vi "правый верхний(SubVI).vi"(10 "Width":u32, 11 "Height":u32) -> (2 "Numeric":u32, 3 "Numeric 2":u32)   [LabVIEW 2021]
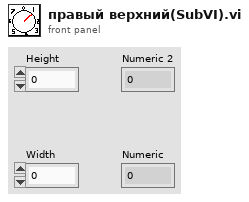
[diagram p1: front panel]
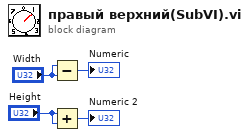
[diagram p0: block diagram]
diagram:
  n1 = Subtract(x="Width", y="Width") -> (x-y=→"Numeric":u32)
  n2 = Add(x="Height", y="Height") -> (x+y=→"Numeric 2":u32)
